vi "Run_Update_Functions0.vi"(3 "Debug Mode":bool, 4 "Time Delta (s)":dbl, 5 "API Function Array":cluster{string, "VI Reference":refnum<vi>}[](array[cluster]), 6 "Update Functions In":cluster{string, string[], dbl[], dbl}[](array[cluster])) -> (0 "Refresh":bool, 1 "Status Array":T1(array[cluster]), 2 "Update Functions Out":cluster{string, string[], dbl[], dbl}[](array[cluster]))   [LabVIEW 2011]
doc: "This VI will execute the appropriate dynamic API VI of all currently running functions during the main loop of a growth run. \"Time Delta (s)\" represents the amount of time in seconds since the last call to this VI. \"Status Array\" will output an array of function statuses from the updated functions, along with the appropriate argument lists to allow other SubVI's to determine the source of each status. \"Debug Mode\" disables all external hardware communications."
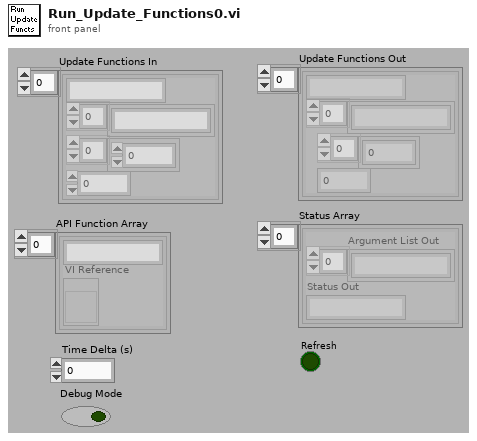
[diagram p1: front panel]
types:
  T1 = cluster{"Argument List Out":string[], "Status Out":string}[]
  T2 = cluster{string, "Argument List Out":string[], dbl[], dbl}
  T3 = enum16{"Discrete", "Continuous", "Instantaneous", "Finite"}
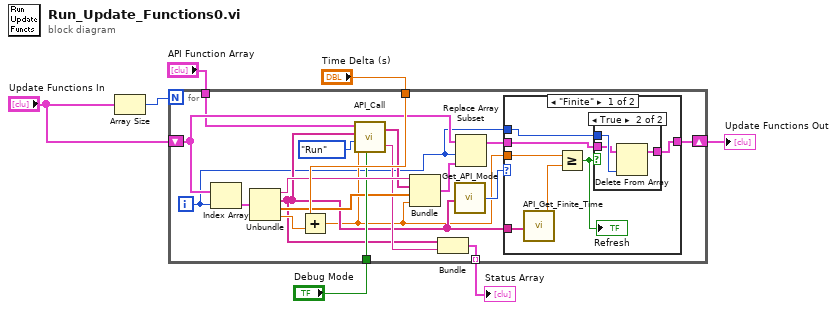
[diagram p0: block diagram]
diagram:
  n1 = Array Size(array="Update Functions In") -> (size(s)=w7:i32)
  n2 = for {
    N: w7 -> [_]
    tunnel: "Time Delta (s)" -> [w25]
    tunnel: "Debug Mode" -> [w20]
    tunnel: [w16] -> w4 mode=indexing
    tunnel: "API Function Array" -> [w15]
    shift-right: [w13] -> w1
    shift-left: "Update Functions In" -> [w22]
    i -> [w8]
    n3 = Index Array(array=w22, index=w8) -> (element=w26:cluster{string, string[], dbl[], dbl})
    n4 = Unbundle(w26) -> (w24:string, w10:string[], w18:dbl[], w19:dbl)
    n5 = Add(x=w25, y=w19) -> (x+y=w9:dbl)
    n6 = call "API_Call.vi"("API Function Array"=w15, "Argument List In"=w10, "State"=enum16{"Edit", "Start", "Run", "End", "Idle"}."Run", "Elapsed Time (s)"=w9, "Debug Mode"=w20) -> ("Argument List Out"=w14:string[], "Status Out"=w17:string)
    n7 = Bundle(w24, "Argument List Out"=w14, w18, w9) -> (w23:T2)  [unwired: 1 out]
    n8 = Bundle(w10, "Status Out"=w17) -> (w16:cluster{string[], "Status Out":string})  [unwired: 1 out]
    n9 = call "Get_API_Mode.vi"("Argument List"=w10) -> ("API Mode"=w11:T3)
    n10 = Replace Array Subset(array=w22, new element=w23, index=w8) -> (w12:cluster{string, string[], dbl[], dbl}[])
    n11 = case shown="\"Finite\"" w11 {
      tunnel: [w30 w38] -> w13
      tunnel: w12 -> [w31 w38]
      tunnel: w10 -> [w29 _]
      tunnel: w9 -> [w33 _]
      tunnel: w8 -> [w32 _]
      frame "Finite" {
        n12 = call "API_Get_Finite_Time.vi"("Argument List"=w29) -> ("Finite Time"=w28:dbl)
        n13 = Greater Or Equal?(x=w33, y=w28) -> (x >= y?=w27:bool)
        "Refresh" <- w27
        n14 = case shown="True" w27 {
          tunnel: w32 -> [_ w37]
          tunnel: w31 -> [w34 w36]
          tunnel: [w34 w35] -> w30
          frame False {
          }
          frame True {
            n15 = Delete From Array(array=w36, index=w37) -> (array with subset deleted=w35:cluster{string, string[], dbl[], dbl}[])  [unwired: 1 in, 1 out]
          }
        }
      }
      frame Default {
      }
    }
  }
  "Update Functions Out" <- w1
  "Status Array" <- w4
